vi "Hex String to String.vi"(1 "hex string":string) -> (0 "string":string)   [LabVIEW 2013]
doc: "Converts hexadecimal string into normal string."
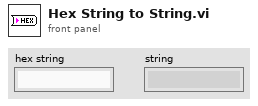
[diagram p1: front panel]
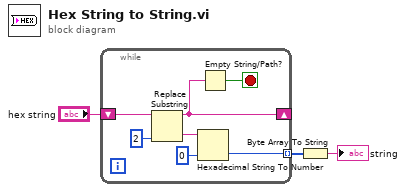
[diagram p0: block diagram]
diagram:
  n1 = while {
    shift-right: [w9] -> _
    shift-left: "hex string" -> [w10]
    tunnel: [w4] -> w2 mode=indexing
    stop <- w8 stop-if-true
    n2 = Replace Substring(2:2 ("length (len. of substring)"), 5:w10) -> (0:w6:string, 1:w9:string)  [unwired: 2 in]
    n3 = Hexadecimal String To Number(string=w6, default (0uL)=u8 0 ("default (0 U32)")) -> (number=w4:u8)  [unwired: 1 in, 1 out]
    n4 = Empty String/Path?(string/path=w9) -> (empty?=w8:bool)
  }
  n5 = Byte Array To String(unsigned byte array=w2) -> (string=→"string":string)
